vi "demo.vi"() -> ()   [LabVIEW 2013]
uses:
  errors/context.ctl
  errors/exception.ctl
  errors/severity.ctl
  errors/error groups/files/file error.ctl
  <vilib>/Utility/VariantDataType/GetTypeInfo.vi
  errors/Variant Repository/Write Variant Repository/Write Exception Property.xnode
  errors/exception.lvlib
  <vilib>/Utility/VariantDataType/VariantType.lvlib
  errors/error groups/files/file errors.lvlib
panel:
  out "exception out 2":T1 {"code" format="%.0x"}
  out "severity 2":T3
  out "file error 2":T4
  out "file exception? 2":bool
  out "file exception 2":T1 {"code" format="%.0x"}
  out "file exception":T1 {"code" format="%.0x"}
  out "file exception?":bool
  out "file error":T4
  out "severity":T3
  out "exception out":T1 {"code" format="%.0x"}
  in  "delay":dbl=10.0 format="%#_13g"
  in  "friendly":bool
  in  "context":T2
  out "text":string
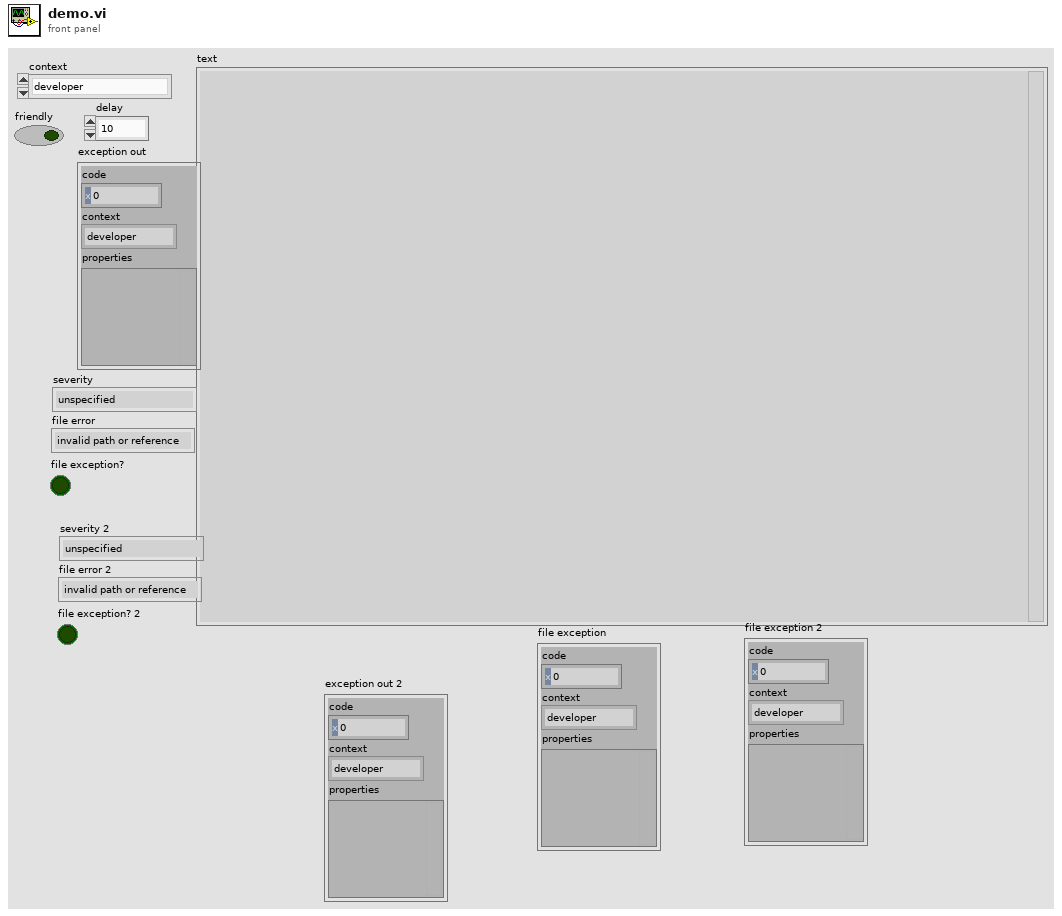
[diagram p1: front panel]
types:
  T1 = typedef "exception.lvlib/exception.ctl" = cluster{"code":i32, "context":T2, "properties":variant}
  T2 = typedef "exception.lvlib/context.ctl" = enum16{"developer", "user interface", "standard", "limited", "deterministic"}
  T3 = typedef "exception.lvlib/severity.ctl" = enum8{"unspecified", "informational", "operation failed", "data corruption", "system corruption", "critical unknown state"}
  T4 = typedef "file errors.lvlib/file error.ctl" = enum16{"invalid path or reference", "end of file", "file already opened", "generic file error", "file not found", "permissions invalid", "disk full", "duplicate path", "too many open file handles", "useless generic error"}
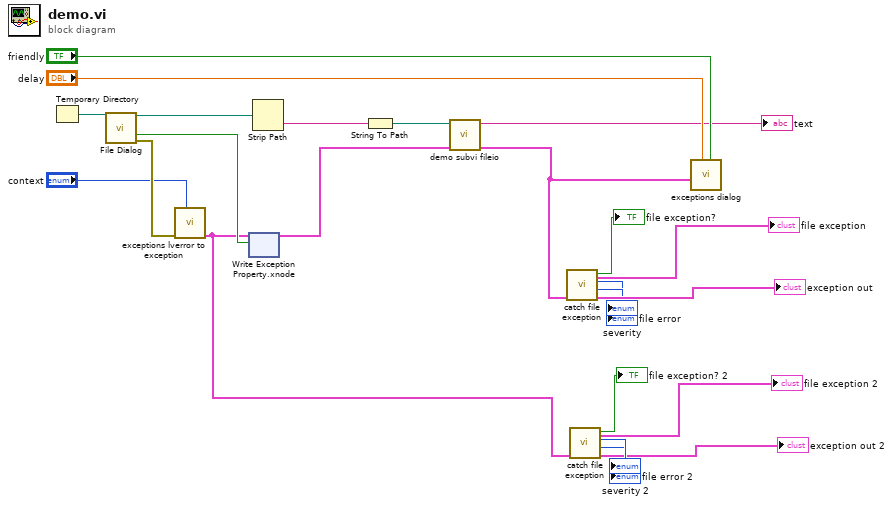
[diagram p0: block diagram]
diagram:
  n1 = Temporary Directory() -> (w16:path)
  n2 = call "File Dialog"("start path"=w16) -> ("selected path"=w21:path, "cancelled"=w13:bool, "error out"=w23:errorcluster)  [unwired: 11 in, 1 out]
  n3 = call "exceptions lverror to exception.vi"("context"="context", "error in"=w23) -> ("exception"=w1:T1)  [unwired: 9 in]
  n4 = xnode "Write Exception Property.xnode"("exception in"=w1, "Value"=w13) -> ("exception out"=w14:T1)  [unwired: 1 in, 1 out]
  n5 = Strip Path(path=w21) -> (name=w20:string)  [unwired: 1 out]
  n6 = String To Path(string=w20) -> (path=w19:path)
  n7 = call "demo subvi fileio.vi"("exception in"=w14, "file path"=w19) -> ("exception out"=w12:T1, "text"=→"text":string)  [unwired: 8 in]
  n8 = call "catch file exception.vi"("exception in"=w12) -> ("exception out"=→"exception out":T1, "severity"=→"severity":T3, "file error"=→"file error":T4, "file exception?"=→"file exception?":bool, "file exception"=→"file exception":T1)  [unwired: 6 in]
  n9 = call "catch file exception.vi"("exception in"=w1) -> ("exception out"=→"exception out 2":T1, "severity"=→"severity 2":T3, "file error"=→"file error 2":T4, "file exception?"=→"file exception? 2":bool, "file exception"=→"file exception 2":T1)  [unwired: 6 in]
  n10 = call "exceptions dialog.vi"("friendly"="friendly", "delay"="delay", "exception"=w12) -> ()  [unwired: 9 in]
